vi "Create Custom Filter.vi"(8 "error in (no error)":errorcluster) -> (0 "error out":errorcluster, 3 "Custom Channel Alias Filter":refnum<k24>)   [LabVIEW 2012]
uses:
  NationalInstruments.VeriStand.SystemStorage
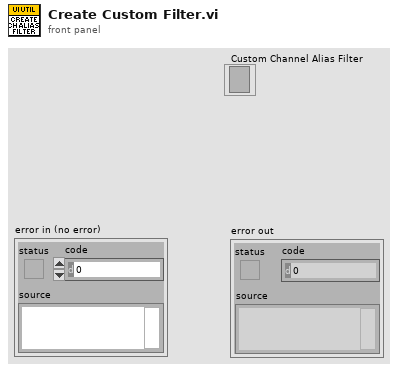
[diagram p1: front panel]
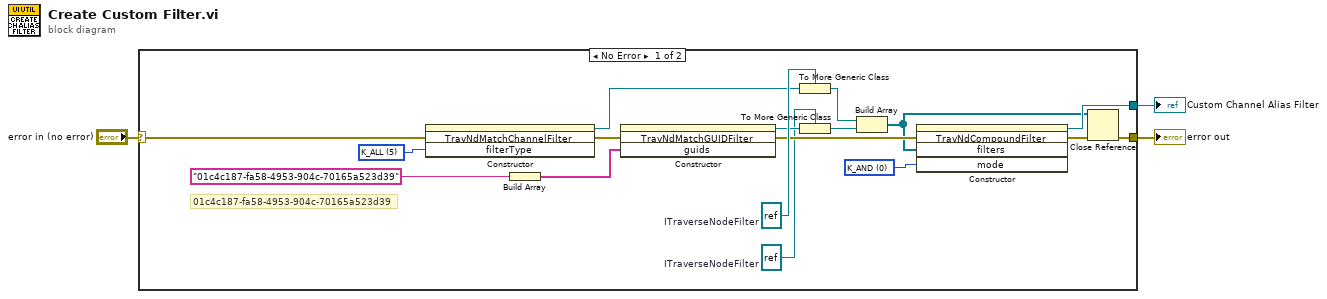
[diagram p0: block diagram]
diagram:
  n1 = case shown="No Error" "error in (no error)" {
    selector: "error in (no error)" -> [w16 w21]
    tunnel: [w19 w21] -> w3
    tunnel: [w17 _] -> w1
    frame No Error {
      w6 = refnum<k24> refnum  # ITraverseNodeFilter
      w12 = 0 items=["K_AND", "K_OR"] ("mode")
      w15 = u8 5 items=["K_CHAN_R", "K_CHAN_W", "K_CHAN_RW", "K_CHAN_VOLT", "K_CHAN_FAULT", "K_ALL", "K_CUSTOM", "K_CHAN_R_VIS", "K_CHAN_W_VIS", "K_CHAN_RW_VIS", "K_CHAN_VOLT_VIS", "K_CHAN_FAULT_VIS", "K_WAVE", "K_WAVE_VIS", "K_WAVE_DBL", "K_WAVE_CDB", "K_WAVE_DBL_VIS", "K_WAVE_CDB_VIS"] ("DisplayFilter")
      w20 = refnum<k24> refnum  # ITraverseNodeFilter
      # "01c4c187-fa58-4953-904c-70165a523d39"
      n2 = constructor class="TravNdMatchChannelFilter"(error in=w16, "filterType"=w15) -> (reference out=w18:refnum<k24>, error out=w13:errorcluster)  [unwired: 2 in, 2 out]
      n3 = Build Array("01c4c187-fa58-4953-904c-70165a523d39") -> (w4:string[])
      n4 = constructor class="TravNdMatchGUIDFilter"(error in=w13, "guids"=w4) -> (reference out=w10:refnum<k24>, error out=w11:errorcluster)  [unwired: 2 in, 2 out]
      n5 = To More Generic Class(target class=w20, reference=w18) -> (generic class reference=w14:refnum<k24>)
      n6 = To More Generic Class(target class=w6, reference=w10) -> (generic class reference=w9:refnum<k24>)
      n7 = Build Array(w14, w9) -> (w7:refnum<k24>[])
      n8 = constructor class="TravNdCompoundFilter"(error in=w11, "filters"=w7, "mode"=w12) -> (reference out=w17:refnum<k24>, error out=w8:errorcluster)  [unwired: 2 in, 3 out]
      n9 = Close Reference(reference=w7, error in (no error)=w8) -> (error out=w19:errorcluster)
    }
    frame Error {
    }
  }
  "error out" <- w3
  "Custom Channel Alias Filter" <- w1
